vi "pointer.allocate random byte array.vi"(8 "error in (no error)":errorcluster, 11 "Pointer in":refnum<class "Memory.Pointer.lvclass">) -> (0 "error out":errorcluster, 2 "random byte array":u8[](array[numeric]), 3 "Pointer out":refnum<class "Memory.Pointer.lvclass">)   [LabVIEW 2016, in "TestCase.Pointer.lvclass"]
uses:
  TestCase.Pointer.lvclass
  Source/Classes/Pointer/Memory.Pointer.lvclass
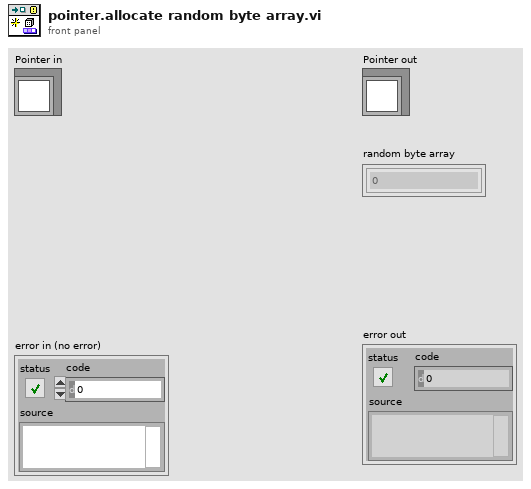
[diagram p1: front panel]
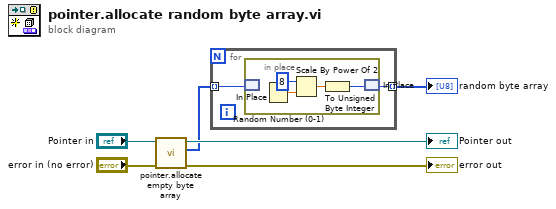
[diagram p0: block diagram]
diagram:
  n1 = call "pointer.allocate empty byte array.vi"("error in (no error)"="error in (no error)", "Pointer in"="Pointer in") -> ("error out"=→"error out":errorcluster, "empty byte array"=w2:u8[], "Pointer out"=→"Pointer out":refnum<class "Memory.Pointer.lvclass">)  [unwired: 7 in]
  n2 = for {
    tunnel: w2 -> [w8] mode=indexing
    tunnel: [w7] -> w1 mode=indexing
    n3 = in-place {
      n4 = in-place-match #1(w8) -> ()  [unwired: 1 out]
      n5 = Random Number (0-1)() -> (number: 0 to 1=w10:dbl)
      n6 = Scale By Power Of 2(n=i16 8, x=w10) -> (x*2^n=w12:dbl)
      n7 = To Unsigned Byte Integer(number=w12) -> (unsigned 8bit integer=w9:u8)
      n8 = in-place-match #1(w9) -> (w7:u8)
    }
  }
  "random byte array" <- w1
